vi "get channel keys.vi"(11 "data allocations":T1) -> (2 "output subquery":string, 3 "input pk list":string[](array[string]))   [LabVIEW 2014, in "SQLite runtime.lvclass"]
uses:
  SQLite runtime.lvclass
  <vilib>/NI/Tag Bus Module Framework/channel/data tables.ctl
  <vilib>/NI/Tag Bus/dictionary/data dictionary.lvclass
  <vilib>/NI/Tag Bus/dictionary table pair.ctl
  <vilib>/NI/Tag Bus/table/data table.ctl
  <vilib>/NI/Tag Bus/table/data table.lvlib
  <vilib>/NI/Tag Bus/tag bus.lvlib
  <vilib>/NI/Tag Bus Module Framework/channel/TBM channel.lvclass
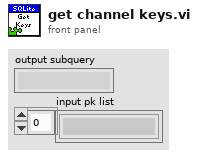
[diagram p1: front panel]
types:
  T1 = typedef "TBM channel.lvclass/data tables.ctl" = cluster{"input data":T2, "processing parameter":T2, "processing result":T2, "output data":T2}
  T2 = typedef "tag bus.lvlib/dictionary table pair.ctl" = cluster{"data dictionary":refnum<class "data dictionary.lvclass">, "data table":T3}
  T3 = typedef "tag bus.lvlib/data table.lvlib/data table.ctl" = cluster{"Double":dbl[], "Single":sgl[], "I64":i64[], "I32":i32[], "I16":i16[], "I8":i8[], "U64":u64[], "U32":u32[], "U16":u16[], "U8":u8[], "Boolean":bool[], "String":string[], "Array of Double":cluster{"DBL Array":dbl[]}[], "Array of Single":cluster{"SGL Array":sgl[]}[], "Array of I64":cluster{"I64 Array":i64[]}[], "Array of I32":cluster{"I32 Array":i32[]}[], "Array of I16":cluster{"I16 Array":i16[]}[], "Array of I8":cluster{"I8 Array":i8[]}[], "Array of U64":cluster{"U64 Array":u64[]}[], "Array of U32":cluster{"U32 Array":u32[]}[], "Array of U16":cluster{"U16 Array":u16[]}[], "Array of U8":cluster{"U8 Array":u8[]}[], "Array of Boolean":cluster{"Boolean Array":bool[]}[], "Array of String":cluster{"String Array":string[]}[]}
  T4 = typedef "tag bus.lvlib/data dictionary.lvclass/full data dictionary.ctl" = cluster{"Double":string[], "Single":string[], "I64":string[], "I32":string[], "I16":string[], "I8":string[], "U64":string[], "U32":string[], "U16":string[], "U8":string[], "Boolean":string[], "String":string[], "Array of Double":string[], "Array of Single":string[], "Array of I64":string[], "Array of I32":string[], "Array of I16":string[], "Array of I8":string[], "Array of U64":string[], "Array of U32":string[], "Array of U16":string[], "Array of U8":string[], "Array of Boolean":string[], "Array of String":string[]}
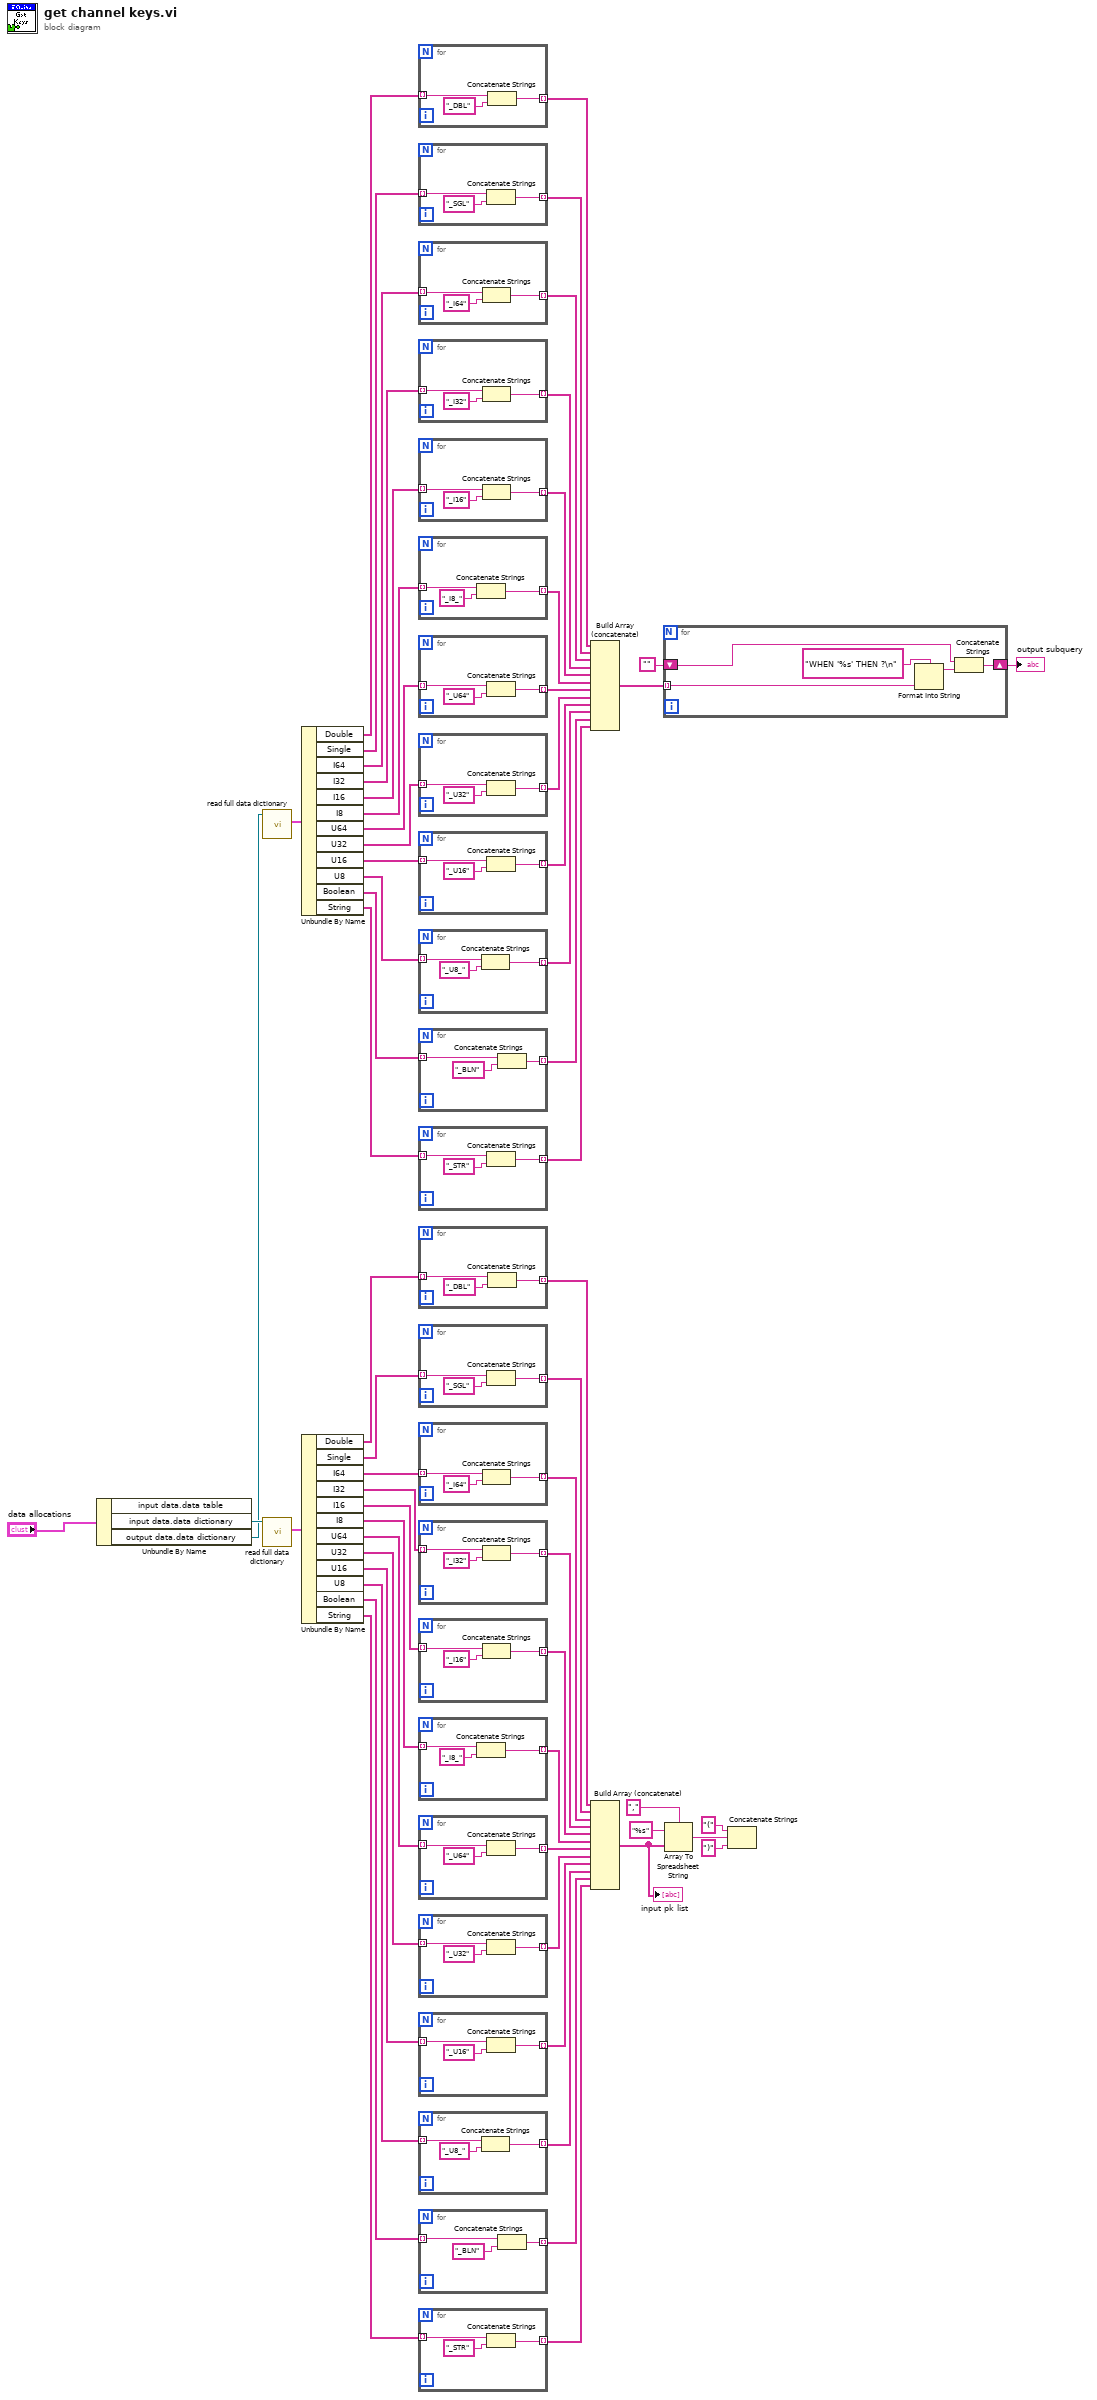
[diagram p0: block diagram]
diagram:
  n1 = Unbundle By Name("data allocations") -> ("input data.data dictionary"=w61:refnum<class "data dictionary.lvclass">, "output data.data dictionary"=w5:refnum<class "data dictionary.lvclass">)  [unwired: 1 out]
  n2 = call <vilib>:"read full data dictionary.vi"("data dictionary in"=w5) -> ("dictionary"=w30:T4)  [unwired: 8 in, 2 out]
  n3 = call <vilib>:"read full data dictionary.vi"("data dictionary in"=w61) -> ("dictionary"=w60:T4)  [unwired: 8 in, 2 out]
  n4 = Unbundle By Name(w30) -> ("Double"=w29:string[], "Single"=w28:string[], "I64"=w27:string[], "I32"=w26:string[], "I16"=w25:string[], "I8"=w24:string[], "U64"=w23:string[], "U32"=w22:string[], "U16"=w21:string[], "U8"=w20:string[], "Boolean"=w19:string[], "String"=w18:string[])
  n5 = Unbundle By Name(w60) -> ("Double"=w59:string[], "Single"=w58:string[], "I64"=w57:string[], "I32"=w56:string[], "I16"=w55:string[], "I8"=w54:string[], "U64"=w53:string[], "U32"=w52:string[], "U16"=w51:string[], "U8"=w50:string[], "Boolean"=w49:string[], "String"=w48:string[])
  n6 = for {
    tunnel: w29 -> [w65] mode=indexing
    tunnel: [w63] -> w17 mode=indexing
    n7 = Concatenate Strings(w65, "_DBL" ("string")) -> (w63:string)
  }
  n8 = for {
    tunnel: w28 -> [w68] mode=indexing
    tunnel: [w66] -> w16 mode=indexing
    n9 = Concatenate Strings(w68, "_SGL" ("string")) -> (w66:string)
  }
  n10 = for {
    tunnel: w27 -> [w71] mode=indexing
    tunnel: [w69] -> w15 mode=indexing
    n11 = Concatenate Strings(w71, "_I64" ("string")) -> (w69:string)
  }
  n12 = for {
    tunnel: w26 -> [w74] mode=indexing
    tunnel: [w72] -> w14 mode=indexing
    n13 = Concatenate Strings(w74, "_I32" ("string")) -> (w72:string)
  }
  n14 = for {
    tunnel: w25 -> [w77] mode=indexing
    tunnel: [w75] -> w13 mode=indexing
    n15 = Concatenate Strings(w77, "_I16" ("string")) -> (w75:string)
  }
  n16 = for {
    tunnel: w24 -> [w80] mode=indexing
    tunnel: [w78] -> w12 mode=indexing
    n17 = Concatenate Strings(w80, "_I8_" ("string")) -> (w78:string)
  }
  n18 = for {
    tunnel: w23 -> [w83] mode=indexing
    tunnel: [w81] -> w11 mode=indexing
    n19 = Concatenate Strings(w83, "_U64" ("string")) -> (w81:string)
  }
  n20 = for {
    tunnel: w22 -> [w86] mode=indexing
    tunnel: [w84] -> w10 mode=indexing
    n21 = Concatenate Strings(w86, "_U32" ("string")) -> (w84:string)
  }
  n22 = for {
    tunnel: w21 -> [w89] mode=indexing
    tunnel: [w87] -> w9 mode=indexing
    n23 = Concatenate Strings(w89, "_U16" ("string")) -> (w87:string)
  }
  n24 = for {
    tunnel: w20 -> [w92] mode=indexing
    tunnel: [w90] -> w8 mode=indexing
    n25 = Concatenate Strings(w92, "_U8_" ("string")) -> (w90:string)
  }
  n26 = for {
    tunnel: w19 -> [w95] mode=indexing
    tunnel: [w93] -> w7 mode=indexing
    n27 = Concatenate Strings(w95, "_BLN" ("string")) -> (w93:string)
  }
  n28 = for {
    tunnel: w18 -> [w98] mode=indexing
    tunnel: [w96] -> w6 mode=indexing
    n29 = Concatenate Strings(w98, "_STR" ("string")) -> (w96:string)
  }
  n30 = for {
    tunnel: w59 -> [w101] mode=indexing
    tunnel: [w99] -> w46 mode=indexing
    n31 = Concatenate Strings(w101, "_DBL" ("string")) -> (w99:string)
  }
  n32 = for {
    tunnel: w58 -> [w104] mode=indexing
    tunnel: [w102] -> w45 mode=indexing
    n33 = Concatenate Strings(w104, "_SGL" ("string")) -> (w102:string)
  }
  n34 = for {
    tunnel: w57 -> [w107] mode=indexing
    tunnel: [w105] -> w44 mode=indexing
    n35 = Concatenate Strings(w107, "_I64" ("string")) -> (w105:string)
  }
  n36 = for {
    tunnel: w56 -> [w110] mode=indexing
    tunnel: [w108] -> w43 mode=indexing
    n37 = Concatenate Strings(w110, "_I32" ("string")) -> (w108:string)
  }
  n38 = for {
    tunnel: w55 -> [w113] mode=indexing
    tunnel: [w111] -> w42 mode=indexing
    n39 = Concatenate Strings(w113, "_I16" ("string")) -> (w111:string)
  }
  n40 = for {
    tunnel: w54 -> [w116] mode=indexing
    tunnel: [w114] -> w41 mode=indexing
    n41 = Concatenate Strings(w116, "_I8_" ("string")) -> (w114:string)
  }
  n42 = for {
    tunnel: w53 -> [w119] mode=indexing
    tunnel: [w117] -> w40 mode=indexing
    n43 = Concatenate Strings(w119, "_U64" ("string")) -> (w117:string)
  }
  n44 = for {
    tunnel: w52 -> [w122] mode=indexing
    tunnel: [w120] -> w39 mode=indexing
    n45 = Concatenate Strings(w122, "_U32" ("string")) -> (w120:string)
  }
  n46 = for {
    tunnel: w51 -> [w125] mode=indexing
    tunnel: [w123] -> w38 mode=indexing
    n47 = Concatenate Strings(w125, "_U16" ("string")) -> (w123:string)
  }
  n48 = for {
    tunnel: w50 -> [w128] mode=indexing
    tunnel: [w126] -> w37 mode=indexing
    n49 = Concatenate Strings(w128, "_U8_" ("string")) -> (w126:string)
  }
  n50 = for {
    tunnel: w49 -> [w131] mode=indexing
    tunnel: [w129] -> w36 mode=indexing
    n51 = Concatenate Strings(w131, "_BLN" ("string")) -> (w129:string)
  }
  n52 = for {
    tunnel: w48 -> [w134] mode=indexing
    tunnel: [w132] -> w35 mode=indexing
    n53 = Concatenate Strings(w134, "_STR" ("string")) -> (w132:string)
  }
  n54 = Build Array (concatenate)(w17, w16, w15, w14, w13, w12, w11, w10, w9, w8, w7, w6) -> (w4:string[])
  n55 = Build Array (concatenate)(w46, w45, w44, w43, w42, w41, w40, w39, w38, w37, w36, w35) -> (w1:string[])
  "input pk list" <- w1
  n56 = for {
    tunnel: w4 -> [w138] mode=indexing
    shift-right: [w137] -> w2
    shift-left: "" -> [w136]
    n57 = Format Into String(format string="WHEN '%s' THEN ?\n", w138) -> (resulting string=w135:string)  [unwired: 2 in, 1 out]
    n58 = Concatenate Strings(w136, w135) -> (w137:string)
  }
  "output subquery" <- w2
  n59 = Array To Spreadsheet String(delimiter (Tab)=",", array=w1, 3:"%s" ("format string")) -> (spreadsheet string=w33:string)
  n60 = Concatenate Strings("(" ("string"), w33, ")" ("string")) -> ()  [unwired: 1 out]
